vi "Msg.vi"(7 "Actor in":refnum<class "Actor.lvclass">, 11 "Actor Destroy Msg Strategy in":refnum<class "Actor Destroy Msg Strategy.lvclass">) -> (0 "error out":errorcluster, 5 "Actor out":refnum<class "Actor.lvclass">)   [LabVIEW 2021, in "Actor Destroy.lvlib" / "Actor Destroy Msg Strategy.lvclass"]
uses:
  Actor Destroy Msg Strategy.lvclass
  LVCAM/Actor/Actor.lvclass
  Actor Destroy/Actor Destroy.lvclass
  be1257ab-8cfd-42d0-bc5a-35db2b78af73.vi
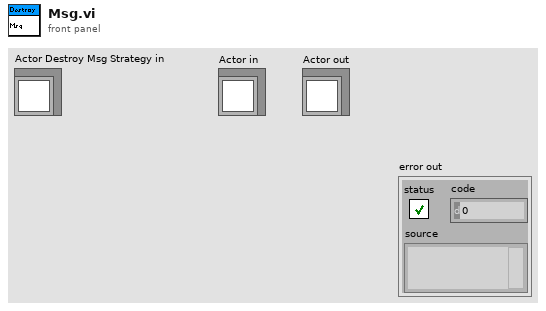
[diagram p1: front panel]
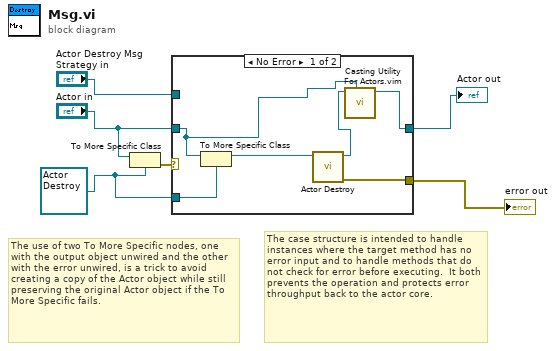
[diagram p0: block diagram]
diagram:
  w1 = refnum<class "Actor Destroy.lvclass"> refnum ("Destroy.lvlib:Destroy.lvclass")
  # "The use of two To More Specific nodes, one with the output object unwired and the other with the error unwired, is a trick to avoid creating a copy of the Actor object while still preserving the original Actor object if the To More Specific fails."
  # "The case structure is intended to handle instances where the target method has no error input and to handle methods that do not check for error before executing.  It both prevents the operation and protects error throughput back to the actor core."
  n1 = To More Specific Class(target class=w1, reference="Actor in") -> (error out=w6:errorcluster)  [unwired: 1 in, 1 out]
  n2 = case shown="No Error" w6 {
    selector: w6 -> [_ w14]
    tunnel: [w12 w14] -> w5
    tunnel: [w7 w13] -> w3
    tunnel: "Actor in" -> [w8 w13]
    tunnel: "Actor Destroy Msg Strategy in" -> [_ _]
    tunnel: w1 -> [w10 _]
    frame No Error {
      n3 = To More Specific Class(target class=w10, reference=w8) -> (specific class reference=w11:refnum<class "Actor Destroy.lvclass">)  [unwired: 1 in, 1 out]
      n4 = call-dynamic "Actor Destroy.vi"("Actor Destroy in"=w11) -> ("error out"=w12:errorcluster, "Actor Destroy out"=w9:refnum<class "Actor Destroy.lvclass">)  [unwired: 9 in]
      n5 = call "Casting Utility For Actors.vim"("type"=w8, "Actor in"=w9) -> ("Actor out"=w7:refnum<class "Actor.lvclass">)  [unwired: 8 in, 1 out]
    }
    frame Error {
      # "If type check fails, pass the original object out again."
    }
  }
  "error out" <- w5
  "Actor out" <- w3
